vi "ep_Read Nominal Frequency.vi"(8 "error in (no error)":errorcluster, 11 "system info in":refnum<class "EP System Info.lvclass">) -> (0 "error out":errorcluster, 1 "nominal frequency value":dbl=50.0, 2 "nominal frequency":enum16{"50 Hz", "60 Hz"}(ring), 3 "system info out":refnum<class "EP System Info.lvclass">)   [LabVIEW 2011, in "NI_EP_Power Quality.lvlib" / "EP System Info.lvclass"]
uses:
  <vilib>/addons/Electrical Power/PQ/Common/Classes/System Info/EP System Info.lvclass
  <vilib>/addons/Electrical Power/PQ/Common/Classes/System Info/EP System Info.lvclass/EP System Info.ctl
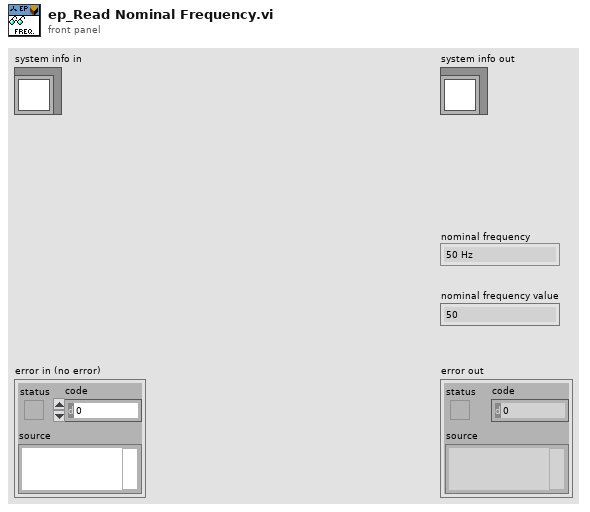
[diagram p1: front panel]
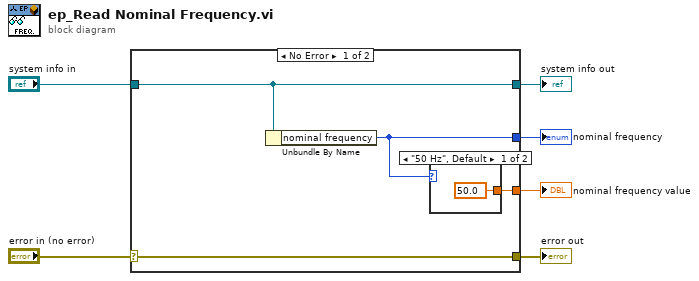
[diagram p0: block diagram]
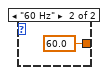
[diagram p2: hidden frame]
diagram:
  n1 = case shown="No Error" "error in (no error)" {
    selector: "error in (no error)" -> [w10 w13]
    tunnel: [w10 w13] -> w5
    tunnel: [w9 w14] -> w3
    tunnel: "system info in" -> [w9 w14]
    tunnel: [w8 _] -> w2
    tunnel: [w7 _] -> w1
    frame No Error {
      n2 = Unbundle By Name(w9) -> ("nominal frequency"=w8:enum16{"50 Hz", "60 Hz"})
      n3 = case shown="\"50 Hz\", Default" w8 {
        tunnel: [50.0 60.0] -> w7
        frame "50 Hz", Default {
        }
        frame "60 Hz" {
        }
      }
    }
    frame Error {
    }
  }
  "error out" <- w5
  "system info out" <- w3
  "nominal frequency" <- w2
  "nominal frequency value" <- w1
